vi "Homing_Z_Stage.vi"(10 "Z Channel ID":i32, 11 "Z Motor":refnum<k7>) -> ()   [LabVIEW 2013]
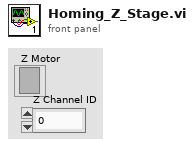
[diagram p1: front panel]
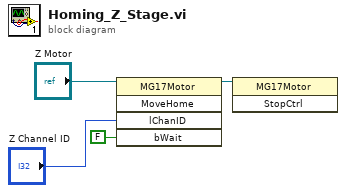
[diagram p0: block diagram]
diagram:
  n1 = invoke class="MG17Motor" method="MoveHome"(reference="Z Motor", "lChanID"="Z Channel ID", "bWait"=FALSE) -> (reference out=w4:refnum<k7>)  [unwired: 2 in, 4 out]
  n2 = invoke class="MG17Motor" method="StopCtrl"(reference=w4) -> ()  [unwired: 2 in, 3 out]
